vi "SubVI_VPdistance_standard.vi"(1 "Basis Object":i32[](array[numeric]), 2 "Test Object":i32[](array[numeric]), 3 "Cost [1/ms]":dbl) -> (0 "VP distance":dbl)   [LabVIEW 2018]
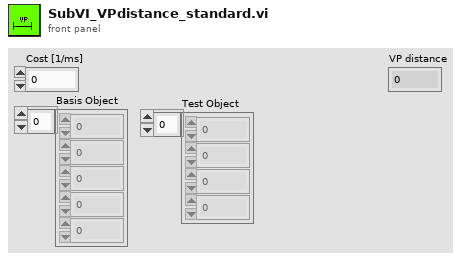
[diagram p1: front panel]
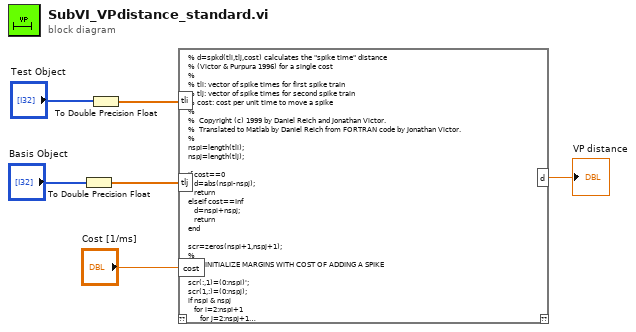
[diagram p0: block diagram]
diagram:
  n1 = To Double Precision Float(number="Basis Object") -> (double precision float=w1:dbl[])
  n2 = To Double Precision Float(number="Test Object") -> (double precision float=w3:dbl[])
  n3 = script code="% d=spkd(tli,tlj,cost) calculates the \"spike time\" distance\n% (Victor & Purpura 1996) for a single cost\n%\n% tli: vector of spike times for first spike train\n% tlj: vector of spike times for second spike train\n% cost: cost per unit time to move a spike\n%\n%  Copyright (c) 1999 by Daniel Reich and Jonathan Victor.\n%  Translated to Matlab by Daniel Reich from FORTRAN code by Jonathan Victor.\n%\nnspi=length(tli);\nnspj=length(tlj);\n\nif cost==0\n   d=abs(nspi-nspj);\n   return\nelseif cost==Inf\n   d=nspi+nspj;\n   return\nend\n\nscr=zeros(nspi+1,nspj+1);\n%\n%     INITIALIZE MARGINS WITH COST OF ADDING A SPIKE\n%\nscr(:,1)=(0:nspi)';\nscr(1,:)=(0:nspj);\nif nspi & nspj\n   for i=2:nspi+1\n      for j=2:nspj+1\n         scr(i,j)=min([scr(i-1,j)+1 scr(i,j-1)+1 scr(i-1,j-1)+cost*abs(tli(i-1)-tlj(j-1))]);\n      end\n   end\nend\nd=scr(nspi+1,nspj+1);" ("Script Node")("tlj"=w1, "tli"=w3, "cost"="Cost [1/ms]") -> ("d"=→"VP distance":dbl)  [unwired: 1 in, 1 out]
